vi "OpticalCamera.vi"() -> ()   [LabVIEW 2025]
panel:
  out "Image Out":T1(plugin-control)
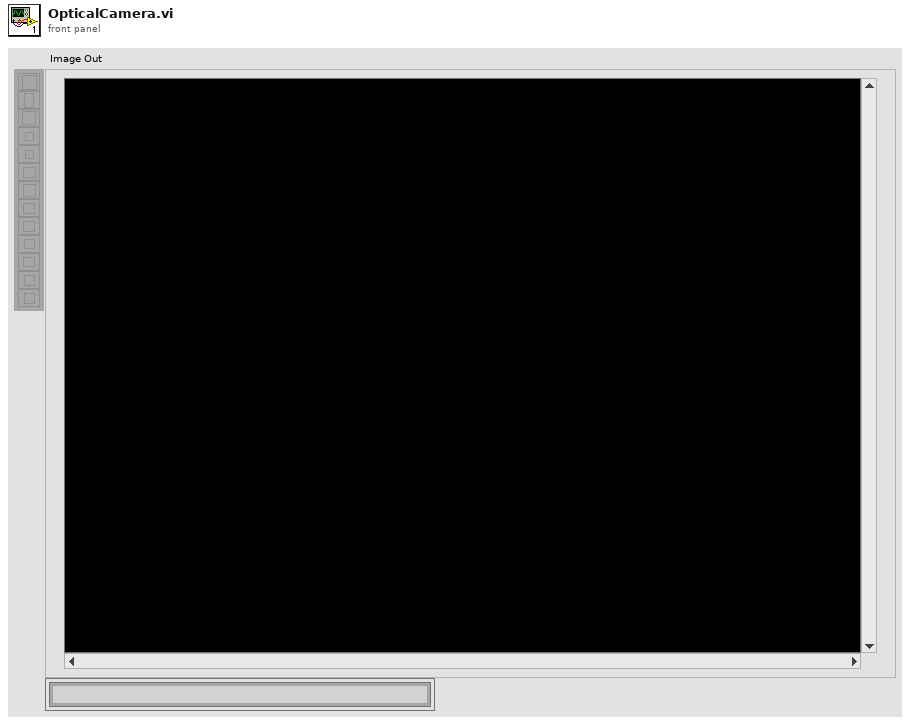
[diagram p1: front panel]
types:
  T1 = typedef "IMAQ Image.ctl" = refnum<image>
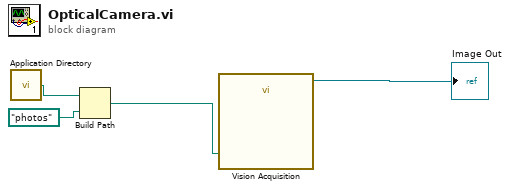
[diagram p0: block diagram]
diagram:
  n1 = call <vilib>:"Application Directory.vi"() -> ("Application Directory"=w3:path)
  n2 = Build Path(base path=w3, name or relative path=path "photos") -> (appended path=w1:path)
  n3 = call "Vision Acquisition"("Image Logging Path"=w1) -> ("Image Out"=→"Image Out":T1)  [unwired: 25 in, 1 out]
